vi "file path property name.vi"() -> (3 "file path property name":string)   [LabVIEW 2017, in "Data Sharing Framework System Explorer.lvlib"]
uses:
  Data Sharing Framework System Explorer.lvlib
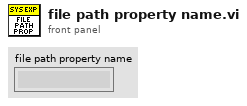
[diagram p1: front panel]
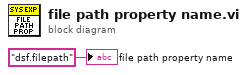
[diagram p0: block diagram]
diagram:
  "file path property name" <- "dsf.filepath" ("Property Name")
